vi "Write_fit_data.vi"(4 "dset name":string, 5 "error in":errorcluster, 6 "fit attribs":variant[](array[variant]), 7 "fit_params":T1(array[cluster]), 8 "ref in":i32) -> (0 "error out":errorcluster, 3 "ref out":i32)   [LabVIEW 2010]
uses:
  <vilib>/addons/h5labview2/attrib/H5Awrite.llb/H5Awrite.xnode
  <vilib>/addons/h5labview2/base/hid_t.ctl
  <vilib>/addons/h5labview2/base/lib_path.vi
  <vilib>/addons/h5labview2/base/H5Equery.vi
  <vilib>/addons/h5labview2/attrib/H5A.lvlib
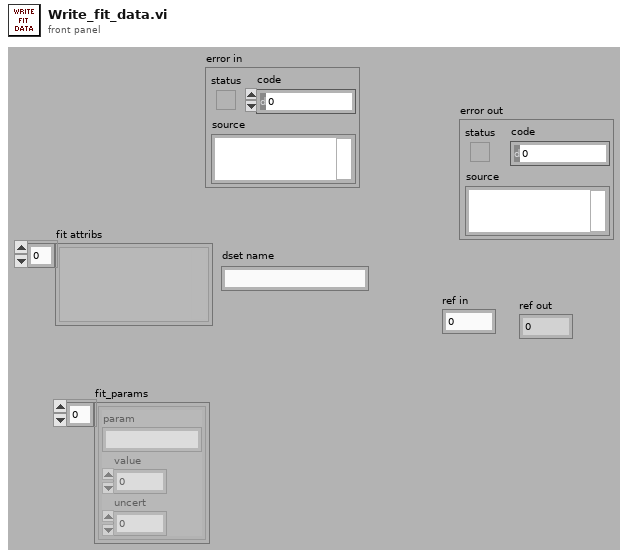
[diagram p1: front panel]
types:
  T1 = cluster{"param":string, "value":dbl, "uncert":dbl}[]
  T2 = typedef "hid_t.ctl" = i32
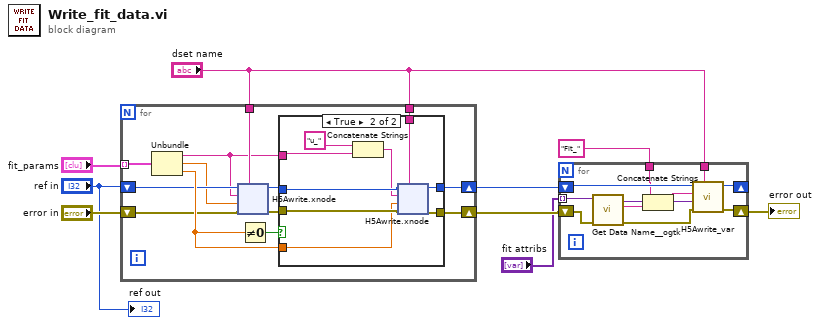
[diagram p0: block diagram]
diagram:
  n1 = for {
    tunnel: "fit_params" -> [w22] mode=indexing
    shift-right: [w18] -> w5
    shift-left: "error in" -> [w14]
    shift-right: [w19] -> w6
    shift-left: "ref in" -> [w13]
    tunnel: "dset name" -> [w12]
    tunnel: "dset name" -> [w17]
    n2 = Unbundle(w22) -> ("param"=w11:string, "value"=w10:dbl, "uncert"=w20:dbl)
    n3 = xnode "H5Awrite.xnode"("object name"=w12, "error in (no error)"=w14, "data"=w10, "attrib name"=w11, "ref in"=w13) -> ("error out"=w15:errorcluster, "ref out"=w16:i32)  [unwired: 2 in, 1 out]
    n4 = Not Equal To 0?(x=w20) -> (x != 0?=w21:bool)
    n5 = case shown="True" w21 {
      tunnel: w15 -> [w41 w46]
      tunnel: w16 -> [w42 w47]
      tunnel: [w42 w48] -> w19
      tunnel: w11 -> [_ w51]
      tunnel: w20 -> [_ w43]
      tunnel: [w41 w49] -> w18
      tunnel: w17 -> [_ w45]
      frame False {
      }
      frame True {
        n6 = Concatenate Strings("u_" ("string"), w51) -> (w44:string)
        n7 = xnode "H5Awrite.xnode"("object name"=w45, "error in (no error)"=w46, "data"=w43, "attrib name"=w44, "ref in"=w47) -> ("error out"=w49:errorcluster, "ref out"=w48:T2)  [unwired: 2 in, 1 out]
      }
    }
  }
  n8 = for {
    tunnel: "fit attribs" -> [w76] mode=indexing
    shift-right: [w80] -> _
    shift-left: w6 -> [w78]
    shift-right: [w79] -> w3
    shift-left: w5 -> [w73]
    tunnel: "dset name" -> [w77]
    tunnel: "Fit_" ("prefix") -> [w70]
    n9 = call <userlib>:"Get Data Name__ogtk.vi"("error in (no error)"=w73, "Data"=w76) -> ("error out"=w72:errorcluster, "Data Name"=w74:string, "Data dup"=w75:variant)  [unwired: 7 in]
    n10 = Concatenate Strings(w70, w74) -> (w71:string)
    n11 = call <vilib>:"H5Awrite_var.vi"("object name"=w77, "error in (no error)"=w72, "data"=w75, "attrib name"=w71, "ref in"=w78) -> ("error out"=w79:errorcluster, "ref out"=w80:T2)  [unwired: 4 in, 1 out]
  }
  "error out" <- w3
  "ref out" <- "ref in"
